vi "CQ2Image.vi"(4 "CQPrams":T2={"Data System params"={"sample freq (MHz)"=50.0, "focal length (mm)"=32.0, "aperature radius (mm)"=3.5, "pts in window"=64.0}, "Show CQ^2 image?"=FALSE, "Save?"=FALSE} {"Data System params"."pts in window" format="%.2f"; "Data System params"."aperature radius (mm)" format="%.2f"; "Data System params"."focal length (mm)" format="%.2f"; "Data System params"."sample freq (MHz)" format="%.2f"}, 5 "name":string, 6 "Tranducer Info":T3 {"start freq" format="%.2f"; "center freq" format="%.2f"; "bandwidth" format="%.2f"}, 7 "midband fit":dbl[][](array[numeric]) format="%.2f", 8 "slope":dbl[][](array[numeric]) format="%.2f", 9 "appended path":path) -> (2 "radius (micron)":sgl[][](graph), 3 "CQ^2":ext[][](graph))   [LabVIEW 2022 SP3]
uses:
  <vilib>/Utility/file.llb/Write Delimited Spreadsheet (DBL).vi
panel:
  in  "material props":T1={"sound speed mm/micros"=1.54, "particle Z"=0.0, "host Zo"=1.0, "scatterer"=0} {"scatterer" items=["isotropic", "cylindrical", "planar"]; "host Zo" format="%.2f"; "particle Z" format="%.2f"; "sound speed mm/micros" format="%.2f"}
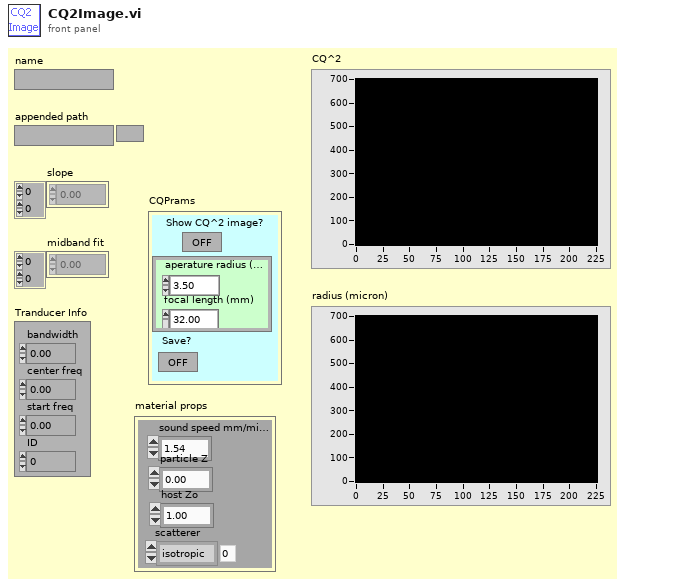
[diagram p1: front panel]
types:
  T1 = cluster{"sound speed mm/micros":dbl, "particle Z":dbl, "host Zo":dbl, "scatterer":i32}
  T2 = cluster{"Data System params":cluster{"sample freq (MHz)":dbl, "focal length (mm)":sgl, "aperature radius (mm)":sgl, "pts in window":dbl}, "Show CQ^2 image?":bool, "Save?":bool}
  T3 = cluster{"bandwidth":sgl, "center freq":sgl, "start freq":sgl, "ID":i32}
  T4 = cluster{"sample freq (MHz)":dbl, "focal length (mm)":sgl, "aperature radius (mm)":sgl, "pts in window":dbl}
  T5 = cluster{"radius (mm)":sgl, "cq^2":ext, "c (part/cc)":ext}
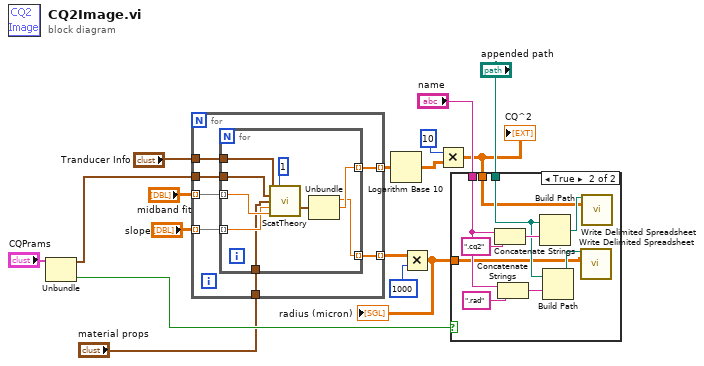
[diagram p0: block diagram]
diagram:
  n1 = Unbundle("CQPrams") -> ("Data System params"=w3:T4, "Save?"=w4:bool)  [unwired: 1 out]
  n2 = for {
    tunnel: "midband fit" -> [w23] mode=indexing
    tunnel: "slope" -> [w22] mode=indexing
    tunnel: "Tranducer Info" -> [w21]
    tunnel: w3 -> [w20]
    tunnel: [w19] -> w11 mode=indexing
    tunnel: [w18] -> w9 mode=indexing
    tunnel: "material props" -> [w17]
    n3 = for {
      tunnel: w23 -> [w32] mode=indexing
      tunnel: w22 -> [w25] mode=indexing
      tunnel: w21 -> [w31]
      tunnel: w20 -> [w30]
      tunnel: [w27] -> w19 mode=indexing
      tunnel: [w26] -> w18 mode=indexing
      tunnel: w17 -> [w24]
      n4 = call "ScatTheory.vi"("Tranducer Info"=w31, "Calc type"=1, "Data System params"=w30, "material props"=w24, "slope"=w25, "midband"=w32) -> ("particle size params"=w28:T5)  [unwired: 2 in, 7 out]
      n5 = Unbundle(w28) -> ("radius (mm)"=w26:sgl, "cq^2"=w27:ext)  [unwired: 1 out]
    }
  }
  n6 = Logarithm Base 10(1:w11) -> (0:w5:ext[][])
  n7 = Multiply(x=w9, y=1000) -> (x*y=w8:sgl[][])
  "radius (micron)" <- w8
  n8 = Multiply(x=10, y=w5) -> (x*y=w6:ext[][])
  "CQ^2" <- w6
  n9 = case shown="True" w4 {
    tunnel: "appended path" -> [_ w36]
    tunnel: "name" -> [_ w37]
    tunnel: w8 -> [_ w33]
    tunnel: w6 -> [_ w34]
    frame False {
    }
    frame True {
      n10 = Concatenate Strings(w37, ".cq2") -> (w42:string)
      n11 = Concatenate Strings(w37, ".rad") -> (w39:string)
      n12 = Build Path(base path=w36, name or relative path=w42) -> (appended path=w40:path)
      n13 = Build Path(base path=w36, name or relative path=w39) -> (appended path=w35:path)
      n14 = call-poly <vilib>:"Write Delimited Spreadsheet.vi"("file path (dialog if empty)"=w35, "2D data"=w33) -> ()  [unwired: 12 in, 2 out]
      n15 = call-poly <vilib>:"Write Delimited Spreadsheet.vi"("file path (dialog if empty)"=w40, "2D data"=w34) -> ()  [unwired: 12 in, 2 out]
    }
  }
